vi "Configure Volume.vi"(5 "Recording Settings":T1, 8 "error in (no error)":errorcluster, 9 "NumReps":i32, 10 "Scan Settings":T2, 11 "AODAcq in":refnum<class "AODAcq.lvclass">) -> (0 "error out":errorcluster, 3 "AODAcq out":refnum<class "AODAcq.lvclass">)   [LabVIEW 2011, in "AODAcq.lvclass"]
uses:
  AODAcq.lvclass
  AODAcq.lvclass/AODAcq.ctl
  <instrlib>/niHWS/nihws.llb/niHWS Write Analog I32.vi
  <vilib>/Utility/error.llb/Error Cluster From Error Code.vi
  Program Files/National Instruments/LabVIEW 2011/Targets/NI/FPGA/StockFPGA_IntfPrivate/ScriptTemplates/StockFPGA_PlugInRead32.vi
  <vilib>/rvi/errors/niLvFpgaAdjustHostInterfaceError.vi
  <vilib>/rvi/interface/nirviReadWriteControl/nirviReadWriteControl.xnode
  FPGA_Control/AODRef.ctl
  FPGA_Control/FPGA Bitfiles/AODControl_FPGATarget_5751Acquire_038F9455.lvbitx
  FPGA_Control/AOD Control (FPGA).vi
  NiFpgaLv.dll
  <vilib>/FPGAPlugInAG/PXIe-7965R/niLvFpga_Read32_PXIe-7965R.vi
  <vilib>/rvi/interface/nirviReadWriteControl/niFpgaRWControlAccessTimeoutTemplate.vi
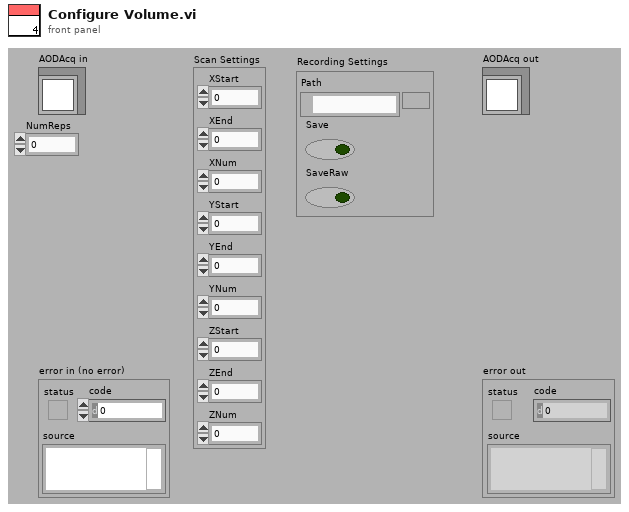
[diagram p1: front panel]
types:
  T1 = cluster{"Path":path, "Save":bool, "SaveRaw":bool}
  T2 = cluster{"XStart":i32, "XEnd":i32, "XNum":i32, "YStart":i32, "YEnd":i32, "YNum":i32, "ZStart":i32, "ZEnd":i32, "ZNum":i32}
  T3 = typedef "AODRef.ctl" = refnum<k20>
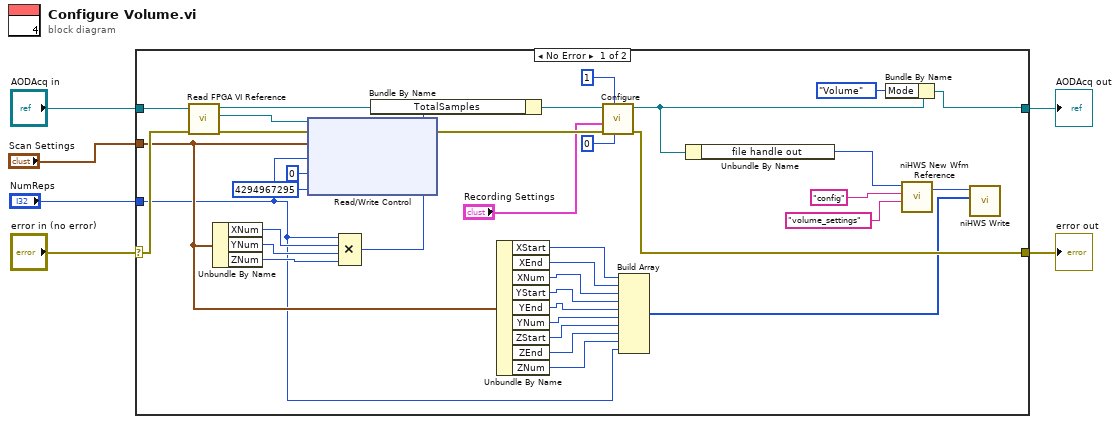
[diagram p0: block diagram]
diagram:
  n1 = case shown="No Error" "error in (no error)" {
    selector: "error in (no error)" -> [w36 w44]
    tunnel: [w35 w44] -> w5
    tunnel: [w10 w43] -> w3
    tunnel: "AODAcq in" -> [w42 w43]
    tunnel: "Scan Settings" -> [w20 _]
    tunnel: "NumReps" -> [w13 _]
    frame No Error {
      n2 = call-dynamic "Read FPGA VI Reference.vi"("error in (no error)"=w36, "AODAcq in"=w42) -> ("error out"=w40:errorcluster, "FPGA VI Reference"=w41:T3, "AODAcq out"=w30:refnum<class "AODAcq.lvclass">)  [unwired: 7 in]
      n3 = Unbundle By Name(w20) -> ("XNum"=w32:i32, "YNum"=w33:i32, "ZNum"=w34:i32)
      n4 = xnode "Read/Write Control"("FPGA VI Reference In"=w41, "error in"=w40, "Scan.VolumeSettings"=w20, "Scan.NumReps"=w13, "Scan.NumMotionPoints"=u32 0, "Scan.Motion Increment"=u32 4294967295) -> ("error out"=w38:errorcluster)  [unwired: 1 out]
      n5 = Compound Arithmetic op=MULTIPLY(w13, w32, w33, w34) -> (w31:i32)
      n6 = Bundle By Name(cluster=w30, "TotalSamples"=w31) -> (w29:refnum<class "AODAcq.lvclass">)
      n7 = Unbundle By Name(w20) -> ("XStart"=w15:i32, "XEnd"=w21:i32, "XNum"=w22:i32, "YStart"=w23:i32, "YEnd"=w24:i32, "YNum"=w25:i32, "ZStart"=w26:i32, "ZEnd"=w27:i32, "ZNum"=w28:i32)
      n8 = call-dynamic "Configure.vi"("GridSize"=u32 0, "Mode"=u32 1, "error in (no error)"=w38, "Recording Settings"="Recording Settings", "AODAcq in"=w29) -> ("error out"=w35:errorcluster, "AODAcq out"=w12:refnum<class "AODAcq.lvclass">)  [unwired: 5 in]
      n9 = Build Array(w15, w21, w22, w23, w24, w25, w26, w27, w28, w13) -> (w14:i32[])
      n10 = Unbundle By Name(w12) -> ("file handle out"=w17:u32)
      n11 = Bundle By Name(cluster=w12, "Mode"=enum16{"Idle", "Points", "Volume"}."Volume") -> (w10:refnum<class "AODAcq.lvclass">)
      n12 = call <instrlib>:"niHWS New Wfm Reference.vi"("waveform name (empty)"="volume_settings", "group name (empty)"="config", "file handle in"=w17) -> ("waveform reference"=w16:u32)  [unwired: 6 in, 2 out]
      n13 = call-poly <instrlib>:"niHWS Write.vi"("data"=w14, "waveform reference in"=w16) -> ()  [unwired: 8 in, 2 out]
    }
    frame Error {
    }
  }
  "error out" <- w5
  "AODAcq out" <- w3
